vi "PJT_07.vi"() -> ()   [LabVIEW 2019]
panel:
  out "A and B":bool
  out "A and B and C":bool
  out "A or B":bool
  in  "C":bool
  in  "B":bool
  in  "A":bool
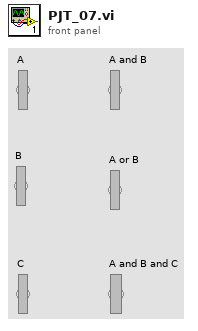
[diagram p1: front panel]
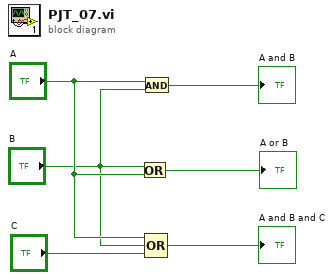
[diagram p0: block diagram]
diagram:
  n1 = Or(x="B", y="A") -> (x .or. y?=→"A or B":bool)
  n2 = And(x="A", y="B") -> (x .and. y?=→"A and B":bool)
  n3 = Compound Arithmetic op=OR ("복합 연산")("A", "B", "C") -> (→"A and B and C":bool)
